vi "filter.vi"() -> ()   [LabVIEW 2009]
panel:
  out "fxp frac":fxp<+/-,16,16>
  in  "in":i16
  in  "stop":bool
  out "fxp":fxp<+/-,16,16>
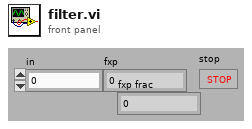
[diagram p1: front panel]
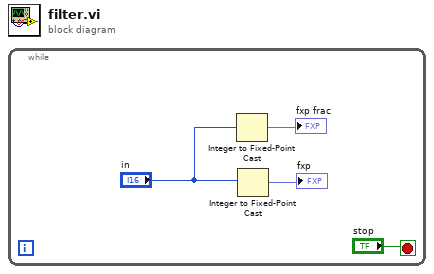
[diagram p0: block diagram]
diagram:
  n1 = while {
    stop <- "stop" stop-if-true
    n2 = Integer to Fixed-Point Cast(integer="in") -> (fixed-point=→"fxp frac":fxp<+/-,16,1>)  [unwired: 1 in]
    n3 = Integer to Fixed-Point Cast(integer="in") -> (fixed-point=→"fxp":fxp<+/-,16,16>)  [unwired: 1 in]
  }
